vi "continuous move simpleV1.2.vi"(8 "error in (no error)":errorcluster, 9 "Position":T1, 10 "Speed":dbl format="%#_13g", 11 "Array":T2) -> (0 "error out":errorcluster, 1 "Position out":T1)   [LabVIEW 2019]
uses:
  move array.ctl
  position cluster.ctl
  <vilib>/Platform/TimedLoop/XDataNode/timing_clust.ctl
  <vilib>/Platform/TimedLoop/XDataNode/nitl_modes.ctl
  <vilib>/Platform/TimedLoop/XDataNode/wakeup.ctl
  <vilib>/myRIO/Instrument Drivers/Onboard IO/DIO/typedefs/DIO Reference.ctl
  <vilib>/myRIO/Common/Instrument Driver Framework/Utilities/typedefs/myRIO Generic Hardware Reference.ctl
  <vilib>/myRIO/Common/Instrument Driver Framework/Utilities/typedefs/Hardware Version Enum.ctl
  <vilib>/myRIO/Common/Instrument Driver Framework/Utilities/typedefs/myRIO v1.0 Reference.ctl
  <vilib>/myRIO/Common/Instrument Driver Framework/Utilities/typedefs/Generic FPGA Reference.ctl
  <vilib>/myRIO/Common/Instrument Driver Framework/myRIO v1.0/DIO/typedefs/DIO Channels List.ctl
  <vilib>/myRIO/Common/Instrument Driver Framework/myRIO v1.0/DIO/typedefs/DIO Channels Enum.ctl
  <vilib>/userDefined/High Color/nirio_resource_hc.ctl
  <vilib>/myRIO/Common/Instrument Driver Framework/Utilities/vis/Is FPGA Ref Available.vi
  <vilib>/myRIO/Common/Instrument Driver Framework/myRIO v1.0/DIO/vis/myRIO v1.1 Open DIO.vi
  <vilib>/myRIO/Instrument Drivers/Onboard IO/DIO/vis/Read.vi
  <vilib>/myRIO/Common/Instrument Driver Framework/Utilities/vis/Validate Channels.vi
  <vilib>/myRIO/Common/Instrument Driver Framework/myRIO v1.0/DIO/vis/myRIO v1.0 Reserve DIO.vi
  <vilib>/myRIO/Common/Instrument Driver Framework/myRIO v1.0/Resource Manager/vis/myRIO v1.0 Reserve Channel List.vi
  <vilib>/myRIO/Common/Instrument Driver Framework/myRIO v1.0/DIO/vis/myRIO v1.0 Build MUX Configuration DIO.vi
  <vilib>/myRIO/Common/Instrument Driver Framework/myRIO v1.0/Resource Manager/vis/myRIO v1.0 Reserve Channel.vi
  <vilib>/myRIO/Common/Instrument Driver Framework/myRIO v1.0/Resource Manager/vis/myRIO v1.0 Unreserve Channel.vi
  <vilib>/myRIO/Common/Instrument Driver Framework/myRIO v1.0/Resource Manager/vis/myRIO v1.0 Create Configuration List.vi
  <vilib>/myRIO/Common/Instrument Driver Framework/myRIO v1.0/Resource Manager/vis/myRIO v1.0 Build Mutex Name.vi
  <vilib>/Utility/VariantDataType/GetNumericInfo.vi
  <vilib>/Utility/error.llb/Error Cluster From Error Code.vi
  <vilib>/myRIO/Common/Instrument Driver Framework/myRIO v1.0/myRIO v1.1 Open.vi
  <vilib>/myRIO/Common/Instrument Driver Framework/Utilities/vis/IO Manager.vi
  <vilib>/myRIO/Common/Instrument Driver Framework/Utilities/vis/Configuration Manager.vi
  <vilib>/myRIO/Common/Instrument Driver Framework/myRIO v1.0/Resource Manager/vis/myRIO v1.0 Configure IO.vi
  <vilib>/myRIO/Common/Instrument Driver Framework/myRIO v1.0/myRIO v1.0 Close.vi
  <vilib>/myRIO/Common/Instrument Driver Framework/myRIO v1.0/DIO/vis/myRIO v1.0 Read DIO.vi
  <vilib>/platform/TimedLoop/XDataNode/XDataNode.xnode
  <vilib>/myRIO/Express VI/Onboard IO/DI/DI Express VI.xnode
  <vilib>/myRIO/Instrument Drivers/Onboard IO/DIO/vis/myRIO DIO Open.xnode
  <vilib>/Platform/TimedLoop/XDataNode/XDNodeRunTimeDep.lvlib
  <vilib>/myRIO/Instrument Drivers/Onboard IO/DIO/DIO.lvlib
panel:
  out "Waveform Chart":dbl(graph)
  out "stop  2":bool
  in  "stop":bool
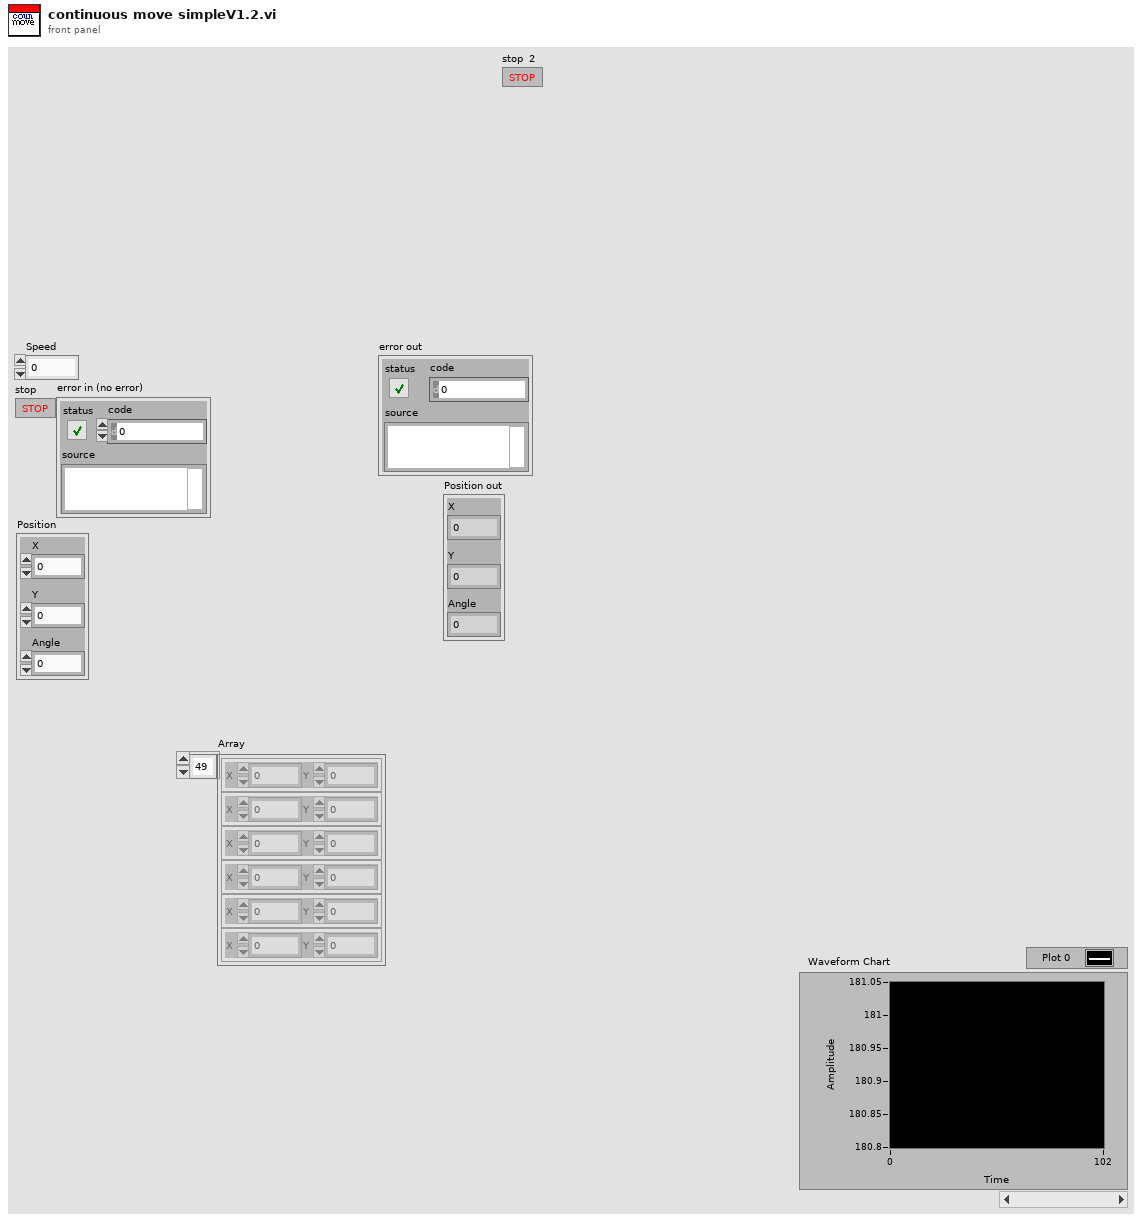
[diagram p1: front panel]
types:
  T1 = typedef "position cluster.ctl" = cluster{"X":dbl, "Y":dbl, "Angle":dbl}
  T2 = typedef "move array.ctl" = cluster{"X":dbl, "Y":dbl}[]
  T3 = typedef "I2C.lvlib/I2C Reference.ctl" = cluster{"myRIO Reference":T4, "I2C Channels Enum":T8, "I2C Configuration":T9}
  T4 = typedef "myRIO Generic Hardware Reference.ctl" = cluster{"myRIO Model":T5, "myRIO Hardware Reference":T6}
  T5 = typedef "Hardware Version Enum.ctl" = enum16{"Unknown", "myRIO-1900", "myRIO-1950", "roboRIO", "NI ELVIS RIO CM", "ELVIS III"}
  T6 = typedef "myRIO v1.0 Reference.ctl" = cluster{"Generic FPGA Reference":T7, "Allow multiple opens":bool}
  T7 = typedef "Generic FPGA Reference.ctl" = refnum<k20>
  T8 = typedef "I2C Channels Enum.ctl" = enum16{"Not Connected", "A/I2C", "B/I2C", "I2C/I2C"}
  T9 = typedef "I2C.lvlib/I2C Configuration.ctl" = cluster{"I2C Transfer Rate":T10}
  T10 = typedef "I2C.lvlib/I2C Transfer Rate.ctl" = enum16{"Standard mode (100 kbps)", "Fast mode (400 kbps)"}
  T11 = typedef "XDNodeRunTimeDep.lvlib/timing_clust.ctl" = cluster{"Expected End [f-1]":u64, "Actual End [f-1]":u64, "Finished Late? [f-1]":bool, "Expected End [i-1]":u64, "Actual End [i-1]":u64, "Finished Late? [i-1]":bool, "Expected Start [i]":u64, "Actual Start [i]":u64, "Expected Start [f]":u64, "Actual Start [f]":u64, "Source Name":string, "Structure Name":string, "Period":i64, "Deadline":i64, "Offset":i64, "Start":i64, "Priority":i32, "Timeout":i32, "Mode":T12, "Wakeup Reason":T13, "Error":errorcluster, "Source Type":string, "Secondary Source Type":string, "Global End Time":u64, "Global Start Time":u64, "Frame Duration":u64, "Iteration Duration":u64, "Assigned CPU":i32, "I/O Scan Engine Mode":u32}
  T12 = typedef "XDNodeRunTimeDep.lvlib/nitl_modes.ctl" = enum32{"No Change", "Process missed periods, maintain original phase", "Discard missed periods, maintain original phase", "Process missed periods, ignore original phase", "Discard missed periods, ignore original phase"}
  T13 = typedef "XDNodeRunTimeDep.lvlib/wakeup.ctl" = enum32{"Normal", "Aborted", "Asynchronous wakeup", "Timing source error", "Timed loop error", "Timeout"}
  T14 = typedef "DIO.lvlib/DIO Reference.ctl" = cluster{"myRIO Reference":T4, "DIO Channels List":T15}
  T15 = typedef "DIO Channels List.ctl" = T16[]
  T16 = typedef "DIO Channels Enum.ctl" = enum16{"Not Connected", "C/DIO0", "C/DIO1", "C/DIO2", "C/DIO3", "C/DIO4", "C/DIO5", "C/DIO6", "C/DIO7", "A/DIO0", "A/DIO1", "A/DIO2", "A/DIO3", "A/DIO4", "A/DIO5", "A/DIO6", "A/DIO7", "A/DIO8", "A/DIO9", "A/DIO10", "A/DIO11", "A/DIO12", "A/DIO13", "A/DIO14", "A/DIO15", "A/DIO16", "A/DIO17", "A/DIO18", "A/DIO19", "B/DIO0", "B/DIO1", "B/DIO2", "B/DIO3", "B/DIO4", "B/DIO5", "B/DIO6", "B/DIO7", "B/DIO8", "B/DIO9", "B/DIO10", "B/DIO11", "B/DIO12", "B/DIO13", "B/DIO14", "B/DIO15", "B/DIO16", "B/DIO17", "B/DIO18", "B/DIO19", "LED0", "LED1", "LED2", "LED3", "Button0", "DIO/DIO0", "DIO/DIO1", "DIO/DIO2", "DIO/DIO3", "DIO/DIO4", "DIO/DIO5", "DIO/DIO6", "DIO/DIO7", "DIO/DIO8", "DIO/DIO9", "SPI/CS0", "SPI/CS1", "SPI/CS2", "SPI/CS3", "LED RADIO (Green)", "LED RADIO (Red)", "LED COMM (Green)", "LED COMM (Red)", "LED MODE (Green)", "LED MODE (Red)"}
  T17 = typedef "nirio_resource_hc.ctl" = tag
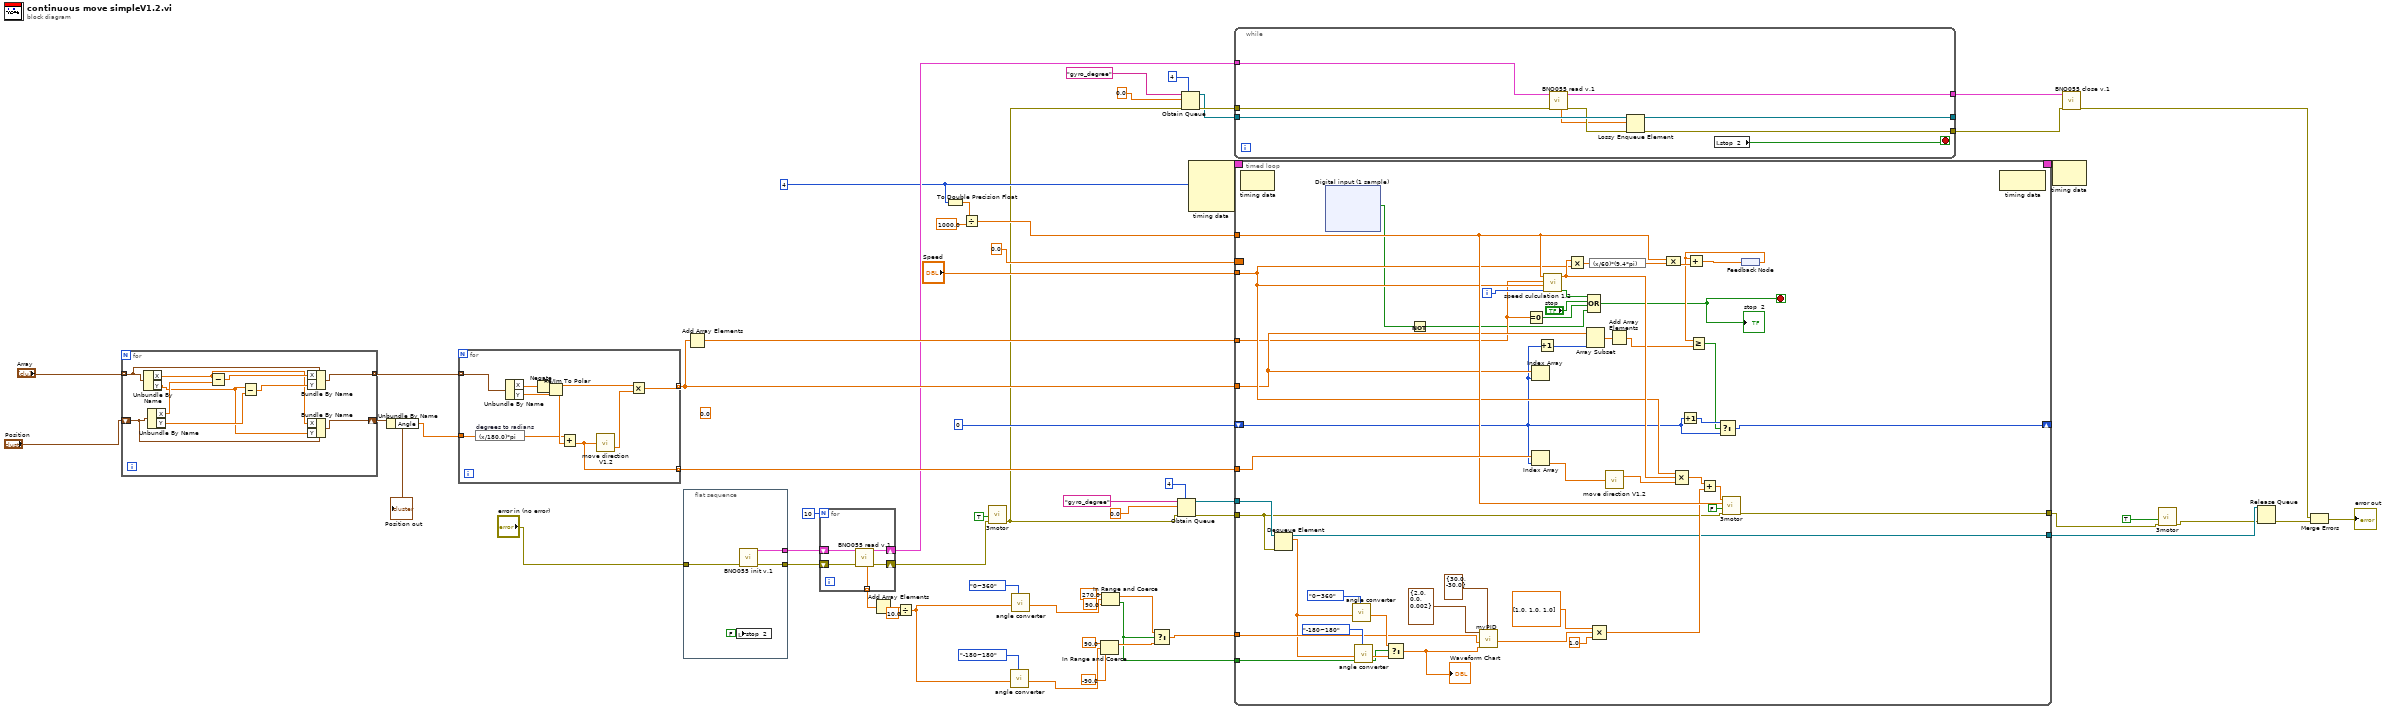
[diagram p0: block diagram]
diagram:
  (unwired) 0.0 ("y")
  w19 = i64 4
  n1 = for {
    tunnel: "Array" -> [w70] mode=indexing
    shift-right: [w62] -> w44
    shift-left: "Position" -> [w65]
    tunnel: [w61] -> w45 mode=indexing
    n2 = Unbundle By Name(w70) -> ("X"=w64:dbl, "Y"=w63:dbl)
    n3 = Unbundle By Name(w65) -> ("X"=w69:dbl, "Y"=w67:dbl)
    n4 = Subtract(x=w64, y=w69) -> (x-y=w68:dbl)
    n5 = Subtract(x=w63, y=w67) -> (x-y=w66:dbl)
    n6 = Bundle By Name(cluster=w70, "X"=w68, "Y"=w66) -> (w61:cluster{"X":dbl, "Y":dbl})
    n7 = Bundle By Name(cluster=w65, "X"=w64, "Y"=w63) -> (w62:T1)
  }
  "Position out" <- w44
  n8 = Unbundle By Name(w44) -> ("Angle"=w43:dbl)
  n9 = for {
    tunnel: w45 -> [w81] mode=indexing
    tunnel: [w77] -> w56 mode=indexing
    tunnel: [w74] -> w57 mode=indexing
    tunnel: w43 -> [w75]
    n10 = expression code="(x/180.0)*pi" "degrees to radians"(w75) -> (w76:dbl)
    n11 = Unbundle By Name(w81) -> ("X"=w80:dbl, "Y"=w79:dbl)
    n12 = Negate(x=w80) -> (-x=w71:dbl)
    n13 = Re/Im To Polar(2:w79, 3:w71) -> (0:w78:dbl, 1:w73:dbl)
    n14 = Add(x=w76, y=w78) -> (x+y=w77:dbl)
    n15 = call "move direction V1.2.vi"("theta"=w77) -> ("max value"=w72:dbl)  [unwired: 1 out]
    n16 = Multiply(x=w73, y=w72) -> (x*y=w74:dbl)
  }
  n17 = flat-sequence {
    tunnel: [w85] -> w41
    tunnel: "error in (no error)" -> [w84]
    tunnel: [w83] -> w42
    frame #0 {
      n18 = local write "stop  2"(FALSE ("stop")) -> ()
      n19 = call "BNO055 init v.1.vi"("error in (no error)"=w84) -> ("error out"=w85:errorcluster, "I2C Ref Out"=w83:T3)  [unwired: 9 in]
    }
  }
  n20 = Add Array Elements(numeric array=w57) -> (sum=w58:dbl)
  n21 = for {
    N: 10 -> [_]
    tunnel: [w87] -> w23 mode=indexing
    shift-right: [w88] -> w40
    shift-left: w42 -> [w90]
    shift-right: [w86] -> w25
    shift-left: w41 -> [w89]
    n22 = call "BNO055 read v.1.vi"("error in (no error)"=w89, "I2C Ref In"=w90) -> ("error out"=w86:errorcluster, "I2C Ref Out"=w88:T3, "degrees out"=w87:dbl)  [unwired: 7 in]
  }
  n23 = Add Array Elements(numeric array=w23) -> (sum=w22:dbl)
  n24 = Divide(x=w22, y=10.0) -> (x/y=w20:dbl)
  n25 = To Double Precision Float(number=w19) -> (double precision float=w53:dbl)
  n26 = Divide(x=w53, y=1000.0) -> (x/y=w51:dbl)
  n27 = call "3motor.vi"("error in (no error)"=w25, "Reset"=TRUE) -> ("error out"=w9:errorcluster)  [unwired: 8 in, 1 out]
  n28 = call "angle converter.vi"("select"=enum16{"-180~180", "0~360"}."-180~180", "input angle"=w20) -> ("angle out"=w37:dbl)  [unwired: 9 in]
  n29 = call "angle converter.vi"("select"=enum16{"-180~180", "0~360"}."0~360", "input angle"=w20) -> ("angle out"=w34:dbl)  [unwired: 9 in]
  n30 = In Range and Coerce(upper limit=90.0, x=w37, lower limit=-90.0) -> (coerced(x)=w30:dbl)  [unwired: 1 out]
  n31 = In Range and Coerce(upper limit=270.0, x=w34, lower limit=90.0) -> (coerced(x)=w31:dbl, In Range?=w28:bool)
  n32 = Select(t=w31, s=w28, f=w30) -> (s? t:f=w27:dbl)
  n33 = Obtain Queue(max queue size (-1, unlimited)=4, name (unnamed)="gyro_degree", element data type=0.0, error in (no error)=w9) -> (queue out=w8:refnum<queue>, error out=w10:errorcluster)  [unwired: 1 in, 1 out]
  n34 = Obtain Queue(max queue size (-1, unlimited)=4, name (unnamed)="gyro_degree", element data type=0.0, error in (no error)=w9) -> (queue out=w14:refnum<queue>, error out=w18:errorcluster)  [unwired: 1 in, 1 out]
  n35 = node-c288(w19) -> (w60:T11)  [unwired: 3 in]
  n36 = while {
    tunnel: w40 -> [w91]
    tunnel: w18 -> [w99]
    tunnel: [w98] -> w26
    tunnel: w14 -> [w97]
    tunnel: [w93] -> w3
    tunnel: [w92] -> _
    stop <- w94 stop-if-true
    n37 = call "BNO055 read v.1.vi"("error in (no error)"=w99, "I2C Ref In"=w91) -> ("error out"=w96:errorcluster, "I2C Ref Out"=w98:T3, "degrees out"=w95:dbl)  [unwired: 7 in]
    n38 = Lossy Enqueue Element(queue=w97, element=w95, error in (no error)=w96) -> (queue out=w92:refnum<queue>, error out=w93:errorcluster)  [unwired: 2 out]
    n39 = local read "stop  2"() -> (w94:bool)
  }
  n40 = timed-loop {
    timing: w60 -> [_]
    timing-out: [_] -> w59
    tunnel: w58 -> [w109]
    tunnel: w57 -> [w128]
    tunnel: w56 -> [w140]
    tunnel: "Speed" -> [w132]
    tunnel: w51 -> [w136]
    border: 0.0 ("y") -> [_]
    shift-right: [w142] -> _
    shift-left: 0 -> [w126]
    tunnel: w10 -> [w106]
    tunnel: [w134] -> w7
    tunnel: w28 -> [w116]
    tunnel: w27 -> [w115]
    tunnel: w8 -> [w107]
    tunnel: [w104] -> w5
    i -> [w147]
    stop <- w102 stop-if-true
    n41 = node-c288() -> ()  [unwired: 1 in, 1 out]
    n42 = Dequeue Element(queue=w107, error in (no error)=w106) -> (queue out=w104:refnum<queue>, element=w105:dbl)  [unwired: 1 in, 2 out]
    n43 = xnode "Digital input (1 sample)"() -> ("A/DIO0 (Pin 11)"=w100:bool)  [unwired: 1 in, 1 out]
    n44 = call "angle converter.vi"("select"=enum16{"-180~180", "0~360"}."0~360", "input angle"=w105) -> ("angle out"=w121:dbl)  [unwired: 9 in]
    n45 = call "angle converter.vi"("select"=enum16{"-180~180", "0~360"}."-180~180", "input angle"=w105) -> ("angle out"=w120:dbl)  [unwired: 9 in]
    n46 = Select(t=w121, s=w116, f=w120) -> (s? t:f=w117:dbl)
    "Waveform Chart" <- w117
    n47 = Not(x=w100) -> (.not. x?=w101:bool)
    n48 = call "myPID.vi"("output range"=cluster{"output high":dbl, "output low":dbl} {"output high"=30.0, "output low"=-30.0}, "Processer"=w117, "setpoint"=w115, "PID"=cluster{"Kp":dbl, "Ki":dbl, "Kd":dbl} {"Kp"=2.0, "Ki"=0.0, "Kd"=0.002}) -> ("out"=w103:dbl)  [unwired: 7 in]
    n49 = Equal To 0?(x=w109) -> (x = 0?=w108:bool)
    n50 = Index Array(array=w128, index=w126) -> ()  [unwired: 1 out]
    n51 = Index Array(array=w140, index=w126) -> (element=w139:dbl)
    n52 = Increment(x=w126) -> (x+1=w127:i32)
    n53 = call "speed culculation 1.2.vi"("i"=w147, "Speed(RPM)"=w132, "distance"=w109, "dt(s)"=w136) -> ("complet?"=w146:bool, "Speed"=w138:dbl)  [unwired: 4 in, 2 out]
    n54 = Multiply(x=w138, y=w132) -> (x*y=w133:dbl)
    n55 = Array Subset(array=w128, length=w127) -> (w129:dbl[])  [unwired: 1 in]
    n56 = Compound Arithmetic op=OR(w146, "stop", w108, w101) -> (w102:bool)
    "stop  2" <- w102
    n57 = expression code="(x/60)*(9.4*pi)"(w133) -> (w144:dbl)
    n58 = Compound Arithmetic op=MULTIPLY(dbl[] [1.0, 1.0, 1.0], w103, 1.0 ("value")) -> (w110:dbl[])
    n59 = call "move direction V1.2.vi"("theta"=w139) -> ("out array"=w137:dbl[])  [unwired: 1 out]
    n60 = Add Array Elements(numeric array=w129) -> (sum=w124:dbl)
    n61 = Compound Arithmetic op=MULTIPLY(w136, w144) -> (w141:dbl)
    n62 = Compound Arithmetic op=MULTIPLY(w132, w138, w137) -> (w111:dbl[])
    n63 = Increment(x=w126) -> (x+1=w143:i32)
    n64 = Add(x=w111, y=w110) -> (x+y=w112:dbl[])
    n65 = call "3motor.vi"("error in (no error)"=w106, "Reset"=FALSE, "dt(s)"=w136, "Motor speed"=w112) -> ("error out"=w134:errorcluster)  [unwired: 6 in, 1 out]
    n66 = feedback #1() -> (w125:dbl)
    n67 = Add(x=w125, y=w141) -> (x+y=w130:dbl)
    n68 = Greater Or Equal?(x=w125, y=w124) -> (x >= y?=w131:bool)
    n69 = Select(t=w143, s=w131, f=w126) -> (s? t:f=w142:i32)
    n70 = feedback-in #1(w130) -> ()
    n71 = node-c288() -> ()  [unwired: 1 in, 1 out]
  }
  n72 = node-c288(w59) -> ()  [unwired: 1 out]
  n73 = call "BNO055 close v.1.vi"("error in (no error)"=w3, "I2C Ref In"=w26) -> ("error out"=w1:errorcluster)  [unwired: 9 in]
  n74 = call "3motor.vi"("error in (no error)"=w7, "Reset"=TRUE) -> ("error out"=w4:errorcluster)  [unwired: 8 in, 1 out]
  n75 = Release Queue(queue=w5, error in (no error)=w4) -> (error out=w6:errorcluster)  [unwired: 1 in, 2 out]
  n76 = Merge Errors(w1, w6) -> (→"error out":errorcluster)
